vi "Class - Friends.vi"(7 "Msg Chain":string, 8 "error in (no error)":errorcluster {"code" format="Error %.0f"}, 10 "Classes":refnum<class "Class Documentation.lvclass">[](array[class]), 11 "VIDoc Printer - Confluence In":refnum<class "VIDoc Printer - Confluence.lvclass">) -> (0 "error out":errorcluster {"code" format="Error %.0f"}, 3 "VIDoc Printer - Confluence Out":refnum<class "VIDoc Printer - Confluence.lvclass">)   [LabVIEW 2023, in "VIDoc Printer - Confluence.lvlib" / "VIDoc Printer - Confluence.lvclass"]
uses:
  VIDoc Printer - Confluence.lvclass
  C:/projects/DMC/Tooling/Git-Action-Service/Source/Documentation Generation/Printers/Printer/VIDoc Printer.lvclass
  Parsing/Class Documentation/Class Documentation.lvclass
  Parsing/Class Documentation/Class Documentation.lvclass/Class Documentation.ctl
  Confluence Formatting/Types/Format Combo Box.ctl
  Parsing/Class Documentation/Get Class_Library.vi
  Parsing/Class Documentation/Get Name.vi
  VIDoc Printer - Confluence.lvclass/VIDoc Printer - Confluence.ctl
  Printer/VIDoc Printer.lvclass
  UI Interaction/UI Interaction.lvclass
  Confluence Formatting/Confluence Formatting.lvlib
  C:/projects/DMC/Tooling/Git-Action-Service/Source/Documentation Generation/Printers/Confluence Printer/VIDoc Printer - Confluence.lvclass
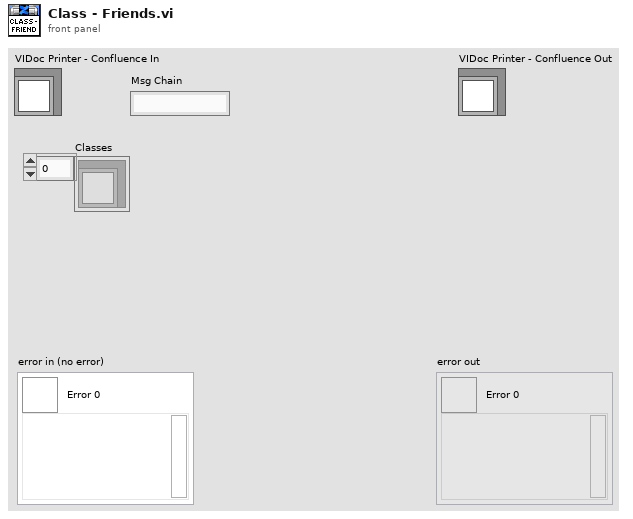
[diagram p1: front panel]
types:
  T1 = typedef "Confluence Formatting.lvlib/Format Combo Box.ctl" = string
  T2 = typedef "VIDoc Parsing.lvlib/Base Class Info Cluster.ctl" = cluster{"Name":string, "Icon":T3, "Version":cluster{"Major":u16, "Minor":u16, "Fix":u16, "Build":u16}, "Description":string, "Friends":string[], "ChildRefsRestricted":bool, "TransferMustOverrides":bool, "Path":path, "Qualified Name":string, "Class Scope":enum32{"invalid scope", "public", "private", "protected", "community"}}
  T3 = typedef "imagedata.ctl" = cluster{"image type":i32, "image depth":i32, "image":u8[], "mask":u8[], "colors":u32[], "Rectangle":cluster{"left":i16, "top":i16, "right":i16, "bottom":i16}}
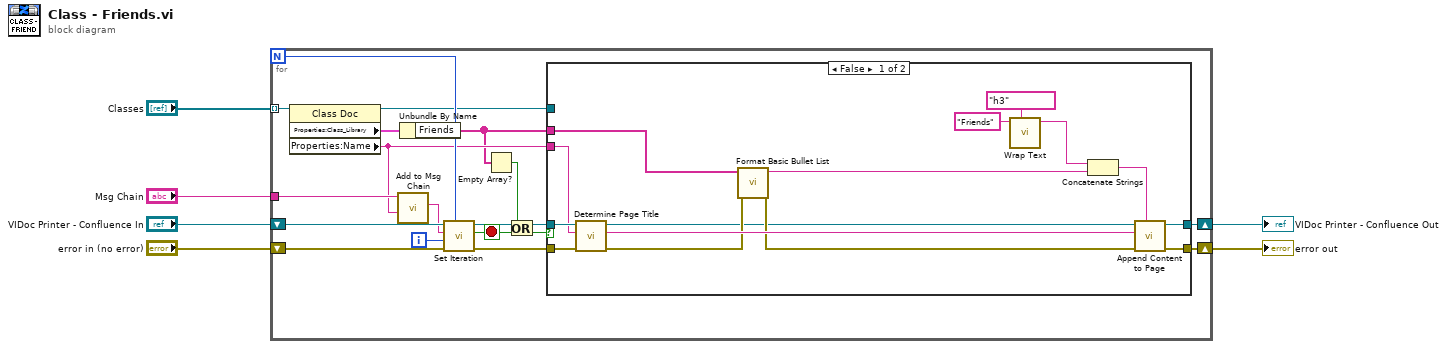
[diagram p0: block diagram]
diagram:
  n1 = for {
    N -> [w17]
    shift-right: [w22] -> w6
    shift-left: "error in (no error)" -> [w20]
    shift-right: [w23] -> w5
    shift-left: "VIDoc Printer - Confluence In" -> [w21]
    tunnel: "Classes" -> [w24] mode=indexing
    tunnel: "Msg Chain" -> [w15]
    i -> [w16]
    stop <- w12 stop-if-true
    n2 = property class="Class Doc"(reference=w24) -> (reference out=w11:refnum<class "Class Documentation.lvclass">, "Properties:Class_Library"=w10:T2, "Properties:Name"=w14:string)  [unwired: 1 in, 1 out]
    n3 = call "Add to Msg Chain.vi"("New"=w14, "Msg Chain in"=w15) -> ("Msg Chain out"=w13:string)  [unwired: 9 in]
    n4 = Unbundle By Name(w10) -> ("Friends"=w9:string[])
    n5 = call "Set Iteration.vi"("Progress Max"=w17, "error in (no error)"=w20, "Progress Value"=w16, "Message (No Message Update)"=w13, "VIDoc Printer In"=w21) -> ("error out"=w18:errorcluster, "Abort?"=w12:bool, "VIDoc Printer Out"=w19:refnum<class "VIDoc Printer - Confluence.lvclass">)  [unwired: 4 in]
    n6 = Empty Array?(array=w9) -> (empty?=w7:bool)
    n7 = Or(x=w7, y=w12) -> (x .or. y?=w8:bool)
    n8 = case shown="False" w8 {
      tunnel: [w38 w40] -> w23
      tunnel: [w37 w41] -> w22
      tunnel: w19 -> [w35 w40]
      tunnel: w18 -> [w34 w41]
      tunnel: w14 -> [w33 _]
      tunnel: w11 -> [_ _]
      tunnel: w9 -> [w25 _]
      frame False {
        n9 = call "Determine Page Title.vi"("error in (no error)"=w34, "Name"=w33, "VIDoc Printer - Confluence In"=w35) -> ("error out"=w29:errorcluster, "Page Title"=w39:string, "VIDoc Printer - Confluence Out"=w27:refnum<class "VIDoc Printer - Confluence.lvclass">)  [unwired: 5 in, 1 out]
        n10 = call "Format Basic Bullet List.vi"("Error in"=w29, "String Array"=w25) -> ("Error out"=w28:errorcluster, "Bullet List"=w26:string)  [unwired: 8 in]
        n11 = call "Wrap Text.vi"("Formatting"=T1 "h3", "String"="Friends") -> ("Wrapped String"=w31:string)  [unwired: 8 in, 1 out]
        n12 = Concatenate Strings(w31, w26) -> (w30:string)
        n13 = call "Append Content to Page.vi"("Page Content"=w30, "error in (no error)"=w28, "Page Title"=w39, "VIDoc Printer - Confluence In"=w27) -> ("error out"=w37:errorcluster, "VIDoc Printer - Confluence Out"=w38:refnum<class "VIDoc Printer - Confluence.lvclass">)  [unwired: 6 in]
      }
      frame True {
      }
    }
  }
  "error out" <- w6
  "VIDoc Printer - Confluence Out" <- w5
